vi "Handle Error.vi"(8 "error in (no error)":errorcluster, 11 "Command Handler in":refnum<class "Command Handler.lvclass">) -> (0 "error out":errorcluster, 2 "stop actor?":bool=TRUE, 3 "Command Handler out":refnum<class "Command Handler.lvclass">)   [LabVIEW 2015, in "Command Handler.lvlib" / "Command Handler.lvclass"]
doc: "(<B>Filename</B>: Actor Framework.lvlib:Actor.lvclass:Handle Error.vi)\n\nDefines how the actor handles an error that occurred while processing a message. By default, this method does nothing except stop the actor."
uses:
  Command Handler.lvclass
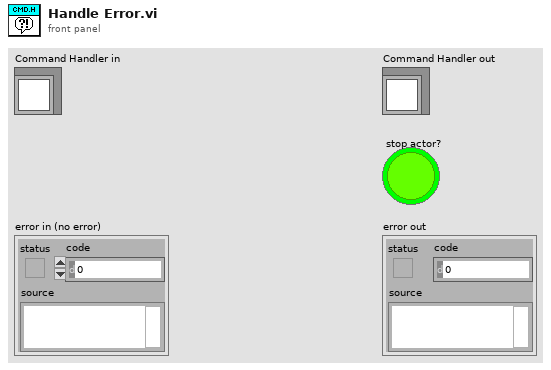
[diagram p1: front panel]
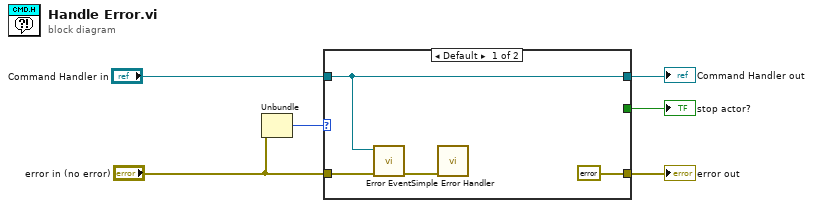
[diagram p0: block diagram]
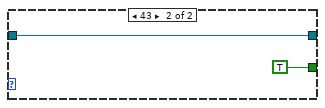
[diagram p2: hidden frame]
diagram:
  n1 = Unbundle("error in (no error)") -> ("code"=w3:i32)  [unwired: 2 out]
  n2 = case shown="Default" w3 {
    tunnel: "Command Handler in" -> [w9 w12]
    tunnel: [w9 w12] -> w6
    tunnel: "error in (no error)" -> [w10 _]
    tunnel: [errorcluster {"status"=FALSE, "code"=0, "source"=""} ("error out") _] -> w5
    tunnel: [_ TRUE ("stop actor?")] -> w4
    frame Default {
      n3 = call "Error Event.vi"("error in (no error)"=w10, "Command Handler in"=w9) -> ("error out"=w7:errorcluster)  [unwired: 9 in]
      n4 = call <vilib>:"Simple Error Handler.vi"("error in (no error)"=w7) -> ()  [unwired: 4 in, 5 out]
    }
    frame 43 {
    }
  }
  "Command Handler out" <- w6
  "error out" <- w5
  "stop actor?" <- w4
